vi "labs.vi"(7 "LabVIEW Web Service Request":refnum<class "Web Request.lvclass">, 11 "context_id":string) -> (3 "labs":T1(array[cluster]))   [LabVIEW 2013]
uses:
  <vilib>/wsapi/Web Request.lvclass
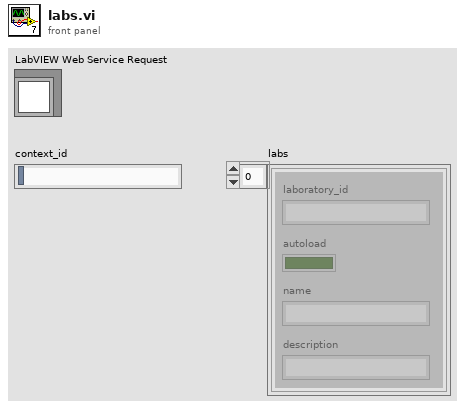
[diagram p1: front panel]
types:
  T1 = cluster{"laboratory_id":string, "autoload":bool, "name":string, "description":string}[]
  T2 = cluster{"laboratory_id":string, "autoload":bool, "name":string, "description":string}
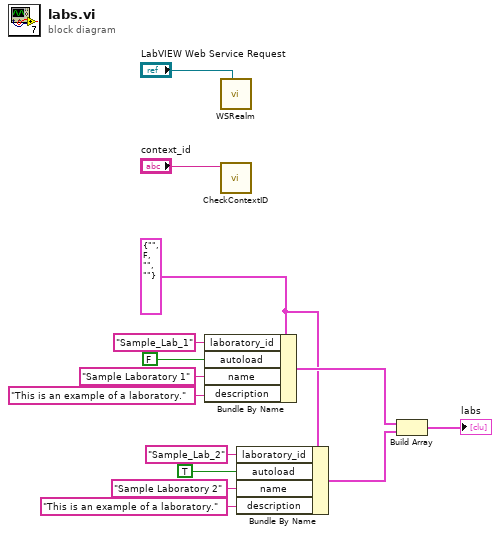
[diagram p0: block diagram]
diagram:
  w9 = T2 {"laboratory_id"="", "autoload"=FALSE, "name"="", "description"=""} ("Cluster")
  n1 = Bundle By Name(cluster=w9, "laboratory_id"="Sample_Lab_1", "autoload"=FALSE, "name"="Sample Laboratory 1", "description"="This is an example of a laboratory.") -> (w11:T2)
  n2 = call "WSRealm.vi"("LabVIEW Web Service Request"="LabVIEW Web Service Request") -> ()  [unwired: 11 in]
  n3 = call "CheckContextID.vi"("context_id"="context_id") -> ()  [unwired: 10 in, 1 out]
  n4 = Bundle By Name(cluster=w9, "laboratory_id"="Sample_Lab_2", "autoload"=TRUE, "name"="Sample Laboratory 2", "description"="This is an example of a laboratory.") -> (w10:T2)
  n5 = Build Array(w11, w10) -> (→"labs":T1)
